vi "Track Generated Frames.vi"(0 "llp packet":T1, 1 "reset":bool, 2 "completed frames register":refnum<k21>, 5 "generate packet":bool, 9 "input valid":bool) -> (14 "ready for input":bool)   [LabVIEW 2020, in "GettingStarted_Gen_148X_FPGA.lvlib"]
uses:
  GettingStarted_Gen_148X_FPGA.lvlib
  <instrlib>/FlexRIO/CSI-2/v2/FPGA/Types/LLP Packet.ctl
  <instrlib>/FlexRIO/CSI-2/v2/FPGA/Types/LLP Packet Header.ctl
  <instrlib>/FlexRIO/CSI-2/v2/FPGA/Types/LLP Packet Payload.ctl
  <instrlib>/FlexRIO/CSI-2/v2/FPGA/Types/LLP Packet Footer.ctl
  <vilib>/rvi/DataTransferAndStorage/Container/Common/niFpgaContainerGetUniqueNameForEmu.vi
  <vilib>/rvi/DataTransferAndStorage/Container/Common/niFpgaContainerSetEmuInfo.vi
  <vilib>/rvi/eio/common/nirviEmuReportErrorAndStop.vi
  <instrlib>/_niInstr/Basic Elements/v1/FPGA/Private/Count Up U32.vi
  <instrlib>/_niInstr/Basic Elements/v1/FPGA/Private/Count Up U16.vi
  <vilib>/rvi/DataTransferAndStorage/Container/Common/niFpgaContainerExecOnDevCompGetState.vi
  <vilib>/rvi/Emulation/niFpgaEmulationIsFPGAContextNoSignature.vi
  <vilib>/rvi/Emulation/niFpgaSctlEmulationGetInTimedLoop.vi
  <vilib>/rvi/errors/niFpgaSetErrorForExecOnDevCompSimple.vi
  <vilib>/rvi/FIFO/Fifo_Resource/nirvififoEmulationSetSize.vi
  <vilib>/rvi/FIFO/Fifo_Resource/nirviFifoEmulationQueueMgr.vi
  <instcachedir>/0/nirviFifoEmulationQueueMgr_E5CAEC123FF24DC58D834DCA3CDAA9B5.lvgen/nirviFifoEmulationQueueMgr_E5CAEC123FF24DC58D834DCA3CDAA9B5_007.vi
  <vilib>/rvi/FIFO/Fifo_Resource/nirvififoEmulationDetermineInputValidOut.vi
  <vilib>/rvi/FIFO/Fifo_Resource/nirvififoEmulationCreateLock.vi
  <vilib>/rvi/Emulation/niFpgaProcessEmulError.vi
  <vilib>/rvi/FIFO/Fifo_Resource/nirvififoEmulationObtainLock.vi
  <vilib>/rvi/FIFO/Fifo_Resource/nirvififoEmulationReleaseLock.vi
  <vilib>/rvi/occurrence/nirviWaitOnOccurrenceBase.vi
  <vilib>/rvi/errors/nirviReportUnexpectedCaseInternalError.vi
  <vilib>/rvi/errors/nirviReportUnexpectedCaseInternalError (U32).vi
  <vilib>/Utility/error.llb/Clear Errors.vi
  <vilib>/rvi/interface/RandomDataEmulation/niFpgaRandomDataHandleErrors.vi
  <vilib>/rvi/Memory/Memory_Emulation/niFpgaMemoryEmulationCacheClearOnFirstRun.vi
  <vilib>/rvi/Memory/Memory_Emulation/nirvimemoryEmulationManagerCache_MakeExclusive.vi
  <vilib>/rvi/Memory/Memory_Emulation/niFpgaMemoryEmulationValidateCache.vi
  <vilib>/rvi/Memory/Memory_Emulation/nirvimemoryEmulationManagerCache_InsertValue.vi
  <vilib>/rvi/Memory/Memory_Emulation/nirvimemoryEmulationManagerCache_ReleaseExclusive.vi
  <vilib>/rvi/Memory/Memory_Emulation/nirvimemoryEmulationManagerCache_GetValue.vi
  <vilib>/rvi/Memory/Memory_Emulation/nirvimemoryEmulationManagerCache_SetValue.vi
  <vilib>/rvi/LocalResourceManager/LocalResourceManager.xnode
  <vilib>/rvi/DataTransferAndStorage/Container/XNode/niFpgaContainer.xnode
  <vilib>/rvi/FIFO/Fifo_Resource/niFpgaFifoEmulationRefIn.vi
  <vilib>/rvi/DataTransferAndStorage/Register/Emulation/niFpgaRegisterEmulationRefIn.vi
  <instrlib>/_niInstr/Basic Elements/v1/FPGA/niInstr Basic Elements v1 FPGA.lvlib
  <instrlib>/FlexRIO/CSI-2/v2/FPGA/NI CSI-2 API FPGA v2.lvlib
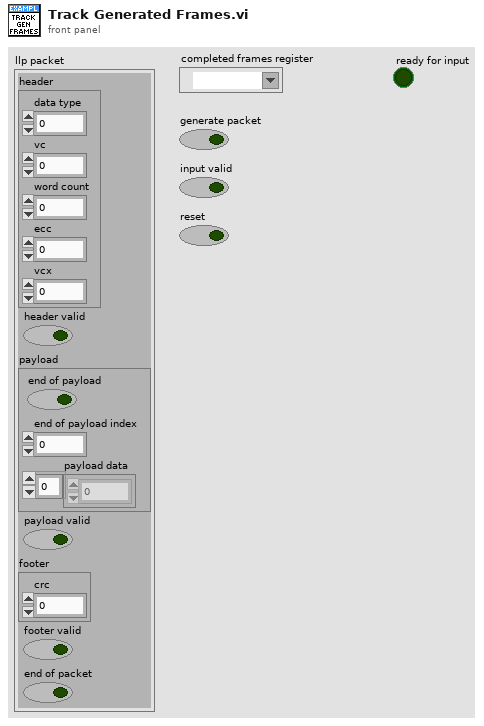
[diagram p1: front panel]
types:
  T1 = typedef "NI CSI-2 API FPGA v2.lvlib/LLP Packet.ctl" = cluster{"header":T2, "header valid":bool, "payload":T3, "payload valid":bool, "footer":T4, "footer valid":bool, "end of packet":bool}
  T2 = typedef "NI CSI-2 API FPGA v2.lvlib/LLP Packet Header.ctl" = cluster{"word count":u16, "ecc":fxp<+,6,6>, "vcx":fxp<+,2,2>, "data type":fxp<+,6,6>, "vc":fxp<+,2,2>}
  T3 = typedef "NI CSI-2 API FPGA v2.lvlib/LLP Packet Payload.ctl" = cluster{"end of payload":bool, "end of payload index":fxp<+,3,3>, "payload data":u8[]}
  T4 = typedef "NI CSI-2 API FPGA v2.lvlib/LLP Packet Footer.ctl" = cluster{"crc":u16}
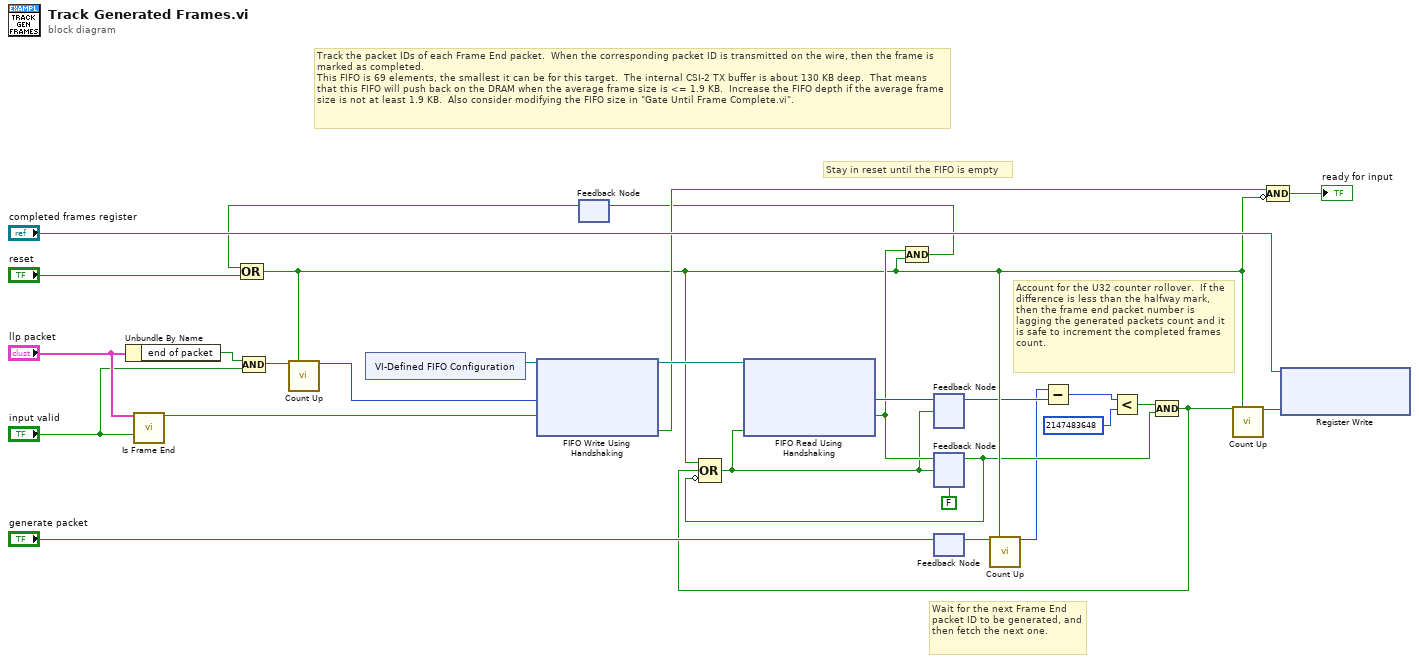
[diagram p0: block diagram]
diagram:
  # "Account for the U32 counter rollover.  If the difference is less than the halfway mark, then the frame end packet number is lagging the generated packets count and it is safe to increment the completed frames count."
  # "Stay in reset until the FIFO is empty"
  # "Wait for the next Frame End  packet ID to be generated, and then fetch the next one."
  # "Track the packet IDs of each Frame End packet.  When the corresponding packet ID is transmitted on the wire, then the frame is marked as completed.\nThis FIFO is 69 elements, the smallest it can be for this target.  The internal CSI-2 TX buffer is about 130 KB deep.  That means that this FIFO will push back on the DRAM when the average frame size is <= 1.9 KB.  Increase the FIFO depth if the average frame size is not at least 1.9 KB.  Also consider modifying the FIFO size in \"Gate Until Frame Complete.vi\"."
  n1 = Unbundle By Name("llp packet") -> ("end of packet"=w19:bool)
  n2 = call <instrlib>:"Is Frame End.vi"("llp packet"="llp packet", "input valid"="input valid") -> ("frame end"=w27:bool)  [unwired: 13 in]
  n3 = Compound Arithmetic op=AND(w19, "input valid") -> (w21:bool)
  n4 = xnode "VI-Defined FIFO Configuration"() -> ("FIFO Out"=w22:refnum<k21>)
  n5 = feedback #1() -> (w17:bool)  [unwired: 1 in]
  n6 = Compound Arithmetic op=OR(w17, "reset") -> (w10:bool)
  n7 = call-poly <instrlib>:"Count Up.vi"("increment"=w21, "reset"=w10) -> ("count out"=w23:u32)  [unwired: 13 in]
  n8 = xnode ("FIFO Write Using Handshaking")("Element"=w23, "Input Valid"=w27, "FIFO In"=w22) -> ("Ready for Input"=w13:bool, "FIFO Out"=w24:refnum<k21>)
  n9 = feedback #2() -> (w3:u32)  [unwired: 1 in]
  n10 = feedback #3(FALSE ("Output Valid")) -> (w7:bool)
  n11 = feedback-in #4("generate packet") -> ()
  n12 = feedback #4() -> (w9:bool)  [unwired: 1 in]
  n13 = call-poly <instrlib>:"Count Up.vi"("increment"=w9, "reset"=w10) -> ("count out"=w2:u32)  [unwired: 13 in]
  n14 = Subtract(x=w2, y=w3) -> (x-y=w1:u32)
  n15 = Less?(x=w1, y=u32 2147483648) -> (x < y?=w4:bool)
  n16 = Compound Arithmetic op=AND(w4, w7) -> (w6:bool)
  n17 = Compound Arithmetic op=OR(w10, w6, invert w7) -> (w14:bool)
  n18 = xnode ("FIFO Read Using Handshaking")("Ready for Output"=w14, "FIFO In"=w24) -> ("Element"=w25:u32, "Output Valid"=w15:bool)  [unwired: 1 out]
  n19 = Compound Arithmetic op=AND(w15, w10) -> (w11:bool)
  n20 = feedback-in #1(w11) -> ()
  n21 = feedback-in #2(w25, w14) -> ()
  n22 = feedback-in #3(w15, w14) -> ()
  n23 = call-poly <instrlib>:"Count Up.vi"("increment"=w6, "reset"=w10) -> ("count out"=w26:u16)  [unwired: 13 in]
  n24 = Compound Arithmetic op=AND(w13, invert w10) -> (→"ready for input":bool)
  n25 = xnode ("Register Write")("Data"=w26, "Register In"="completed frames register") -> ()  [unwired: 1 out]
